vi "Read Unsubscribe Msg.vi"(11 "IObserver in":refnum<class "IObserver.lvclass">) -> (2 "Pre-Addressed Unsubscribe Msg":refnum<class "Unsubscribe Msg.lvclass">)   [LabVIEW 2018, in "MVA Framework.lvlib" / "IObserver.lvlib" / "IObserver.lvclass"]
doc: "读取取消订阅消息"
uses:
  IObserver.lvclass
  IMediator/IMediator Messages/Unsubscribe Msg/Unsubscribe Msg.lvclass
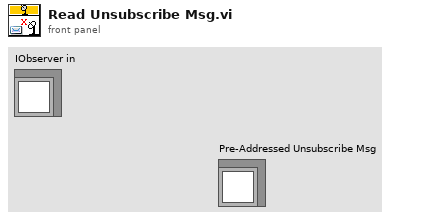
[diagram p1: front panel]
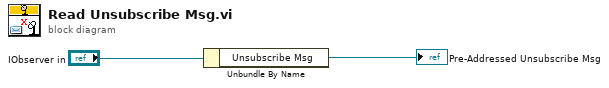
[diagram p0: block diagram]
diagram:
  n1 = Unbundle By Name("IObserver in") -> ("Unsubscribe Msg"=→"Pre-Addressed Unsubscribe Msg":refnum<class "Unsubscribe Msg.lvclass">)
